vi "rinse_FMI.vi"(0 "Prime?":bool=TRUE, 6 "OpenValve#":i32=10, 7 "RequestedValve#":i32) -> ()   [LabVIEW 2019]
panel:
  out "xxx":bool[](array[boolean])
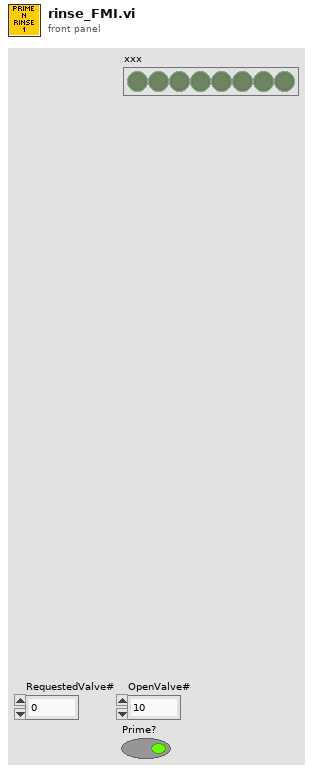
[diagram p1: front panel]
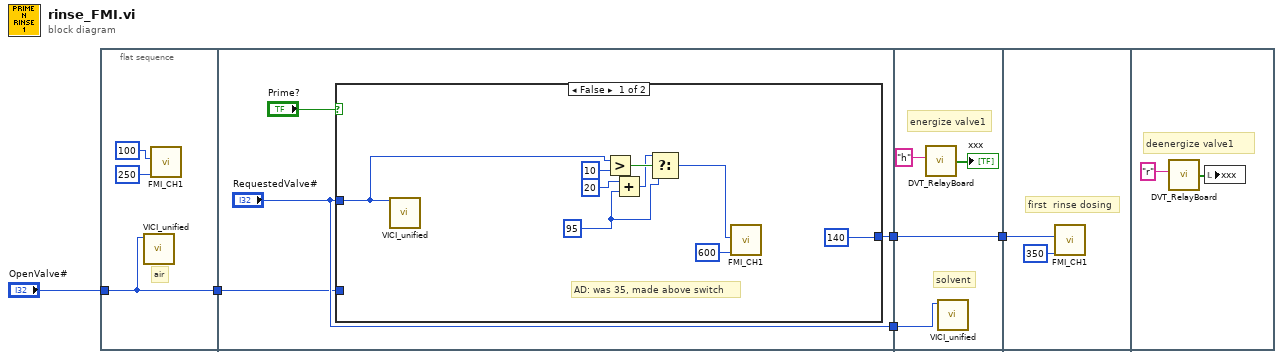
[diagram p0: block diagram]
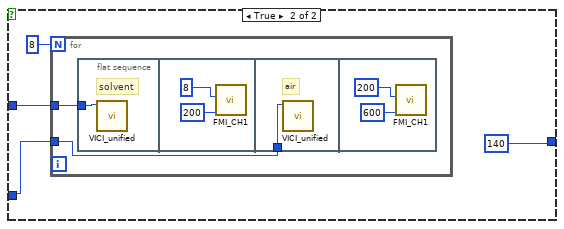
[diagram p2: hidden frame]
diagram:
  n1 = flat-sequence {
    tunnel: "OpenValve#" -> [w8]
    tunnel: [w8] -> w3
    tunnel: ["RequestedValve#"] -> w5
    tunnel: w3 -> [w10]
    tunnel: [w9] -> w1
    tunnel: w5 -> [w37]
    tunnel: [w34] -> w2
    tunnel: w1 -> [w34]
    tunnel: w2 -> [w38]
    frame #0 {
      # "air"
      n2 = call "VICI_unified.vi"("RequestedValve#"=w8) -> ()  [unwired: 11 in]
      n3 = call "FMI_CH1.vi"("RPM"=250, "Strokes"=100) -> ()  [unwired: 6 in]
    }
    frame #1 {
      n4 = case shown="False" "Prime?" {
        tunnel: "RequestedValve#" -> [w16 w23]
        tunnel: w10 -> [_ w24]
        tunnel: [140 ("Strokes") 140 ("Strokes")] -> w9
        frame False {
          w14 = 95 ("Strokes")
          # "AD: was 35, made above switch"
          n5 = call "VICI_unified.vi"("RequestedValve#"=w16) -> ()  [unwired: 11 in]
          n6 = Greater?(x=w16, y=10) -> (0:w19:bool)
          n7 = Add(x=20, y=w14) -> (x+y=w15:i32)
          n8 = Select(t=w15, s=w19, f=w14) -> (s? t:f=w13:i32)
          n9 = call "FMI_CH1.vi"("RPM"=600, "Strokes"=w13) -> ()  [unwired: 6 in]
        }
        frame True {
          n10 = for {
            N: 8 -> [_]
            tunnel: w23 -> [w27]
            tunnel: w24 -> [w26]
            n11 = flat-sequence {
              tunnel: w27 -> [w28]
              tunnel: w26 -> [w31]
              frame #0 {
                # "solvent"
                n12 = call "VICI_unified.vi"("RequestedValve#"=w28) -> ()  [unwired: 11 in]
              }
              frame #1 {
                n13 = call "FMI_CH1.vi"("RPM"=200, "Strokes"=8) -> ()  [unwired: 6 in]
              }
              frame #2 {
                # "air"
                n14 = call "VICI_unified.vi"("RequestedValve#"=w31) -> ()  [unwired: 11 in]
              }
              frame #3 {
                n15 = call "FMI_CH1.vi"("RPM"=600, "Strokes"=200) -> ()  [unwired: 6 in]
              }
            }
          }
        }
      }
    }
    frame #2 {
      # "energize valve1"
      # "solvent"
      n16 = call "DVT_RelayBoard.vi"("write buffer"="h") -> ("Boolean array"=→"xxx":bool[])  [unwired: 3 in, 2 out]
      n17 = call "VICI_unified.vi"("RequestedValve#"=w37) -> ()  [unwired: 11 in]
    }
    frame #3 {
      # "first  rinse dosing"
      n18 = call "FMI_CH1.vi"("RPM"=350, "Strokes"=w38) -> ()  [unwired: 6 in]
    }
    frame #4 {
      # "deenergize valve1"
      n19 = call "DVT_RelayBoard.vi"("write buffer"="r") -> ("Boolean array"=w41:bool[])  [unwired: 3 in, 2 out]
      n20 = local write "xxx"(w41) -> ()
    }
  }
